vi "Get handle or release handle_YCC.vi"() -> ()   [LabVIEW 2014]
uses:
  Main-Stage-PI/(Global) Current handle and LaserPower_YCC.vi
  SubVI-Stage-Based/MCL-dll-Labview 32-bit/Madlib.dll
panel:
  in  "Enum":enum16{"Get current handle", "Release handle"}(ring)
  out "Current handle":i32
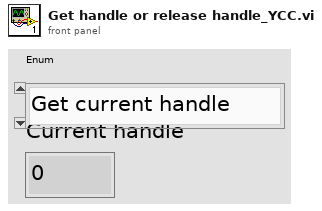
[diagram p1: front panel]
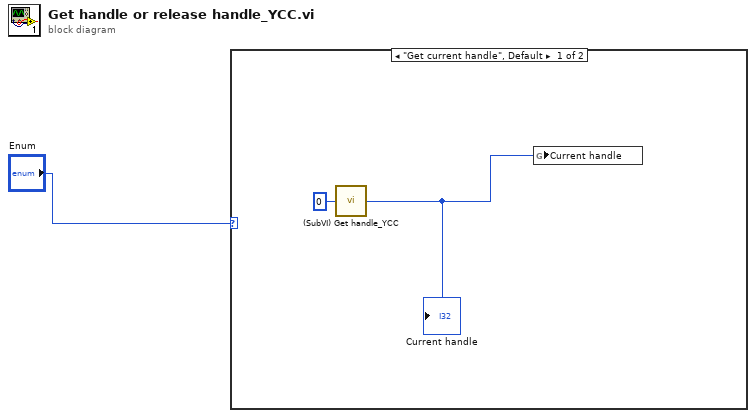
[diagram p0: block diagram]
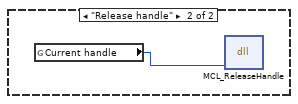
[diagram p2: hidden frame]
diagram:
  n1 = case shown="\"Get current handle\", Default" "Enum" {
    frame "Get current handle", Default {
      n2 = call "(SubVI) Get handle_YCC.vi"("Incoming Handle"=0) -> ("Outgoing Handle"=w2:i32)
      "Current handle" <- w2
      n3 = global write "(Global) Current handle and LaserPower_YCC.vi" "Current handle"(w2) -> ()
    }
    frame "Release handle" {
      n4 = global read "(Global) Current handle and LaserPower_YCC.vi" "Current handle"() -> (w4:i32)
      n5 = dll-call lib="C:/Users/hwlab/OneDrive - g.ntu.edu.tw/OT/YCC's OT-PI/Main-Stage-Based/SubVI-Stage-Based/MCL-dll-Labview 32-bit/MADLib.dll" fn="MCL_ReleaseHandle"("handle"=w4) -> ()  [unwired: 5 in, 2 out]
    }
  }
